vi "MoveAbsSingleAxis.vi"(6 "Wait":bool=TRUE, 8 "error in (no error)":errorcluster caption="entrée d'erreur (pas d'erreur)", 9 "Value":dbl format="%.2f", 10 "Axis":i32=1, 11 "DelayLineLS4 en entrée":refnum<class "DLLS4.lvclass">) -> (0 "error out":errorcluster caption="sortie d'erreur", 3 "DelayLineLS4 en sortie":refnum<class "DLLS4.lvclass">)   [LabVIEW 2015, in "DLLS4.lvclass"]
uses:
  DLLS4.lvclass
  DelayLine.lvclass/DelayLine.ctl
  <vilib>/Utility/error.llb/DialogType.ctl
  DelayLine.lvclass
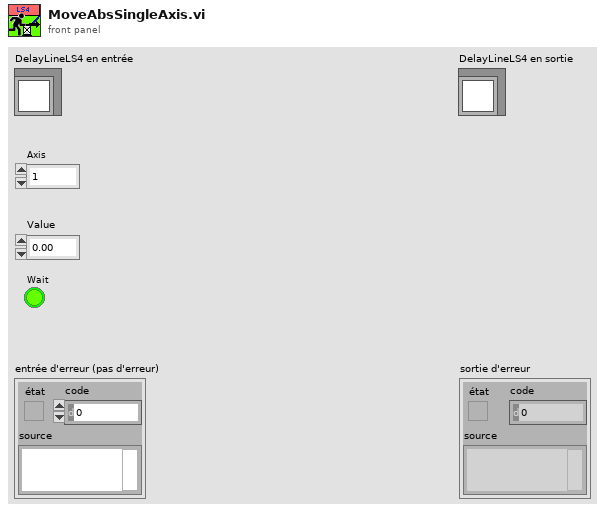
[diagram p1: front panel]
types:
  T1 = typedef "DialogType.ctl" = u16
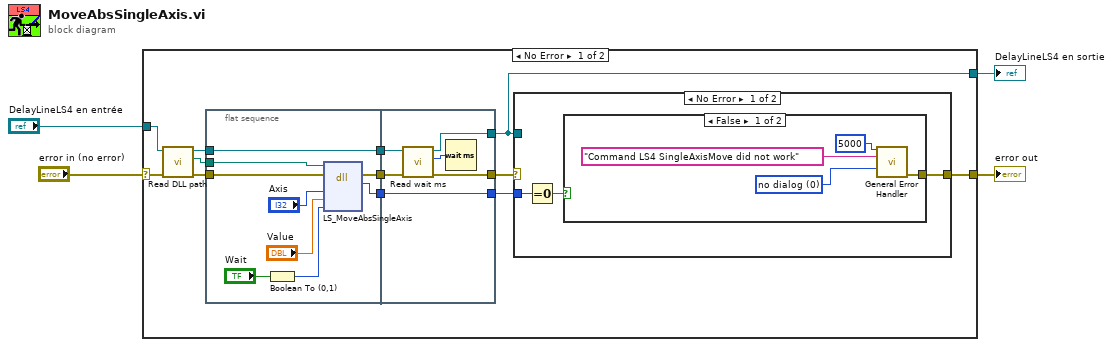
[diagram p0: block diagram]
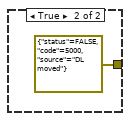
[diagram p2: hidden frame]
diagram:
  n1 = case shown="No Error" "error in (no error)" {
    selector: "error in (no error)" -> [w15 w42]
    tunnel: [w16 w42] -> w2
    tunnel: [w9 w41] -> w1
    tunnel: "DelayLineLS4 en entrée" -> [w12 w41]
    frame No Error {
      n2 = call "Read DLL path.vi"("error in (no error)"=w15, "DelayLine in"=w12) -> ("error out"=w14:errorcluster, "DLL path"=w13:path, "DelayLine out"=w11:refnum<class "DLLS4.lvclass">)  [unwired: 7 in]
      n3 = flat-sequence {
        tunnel: w14 -> [w26]
        tunnel: w13 -> [w30]
        tunnel: w11 -> [w29]
        tunnel: [w29] -> w10
        tunnel: [w28] -> w8
        tunnel: [w27] -> w6
        tunnel: [w37] -> w9
        tunnel: w10 -> [w38]
        tunnel: [w35] -> w7
        tunnel: w8 -> [w39]
        tunnel: [w40] -> w5
        tunnel: w6 -> [w40]
        frame #0 {
          n4 = Boolean To (0,1)(Boolean="Wait") -> (0, 1=w32:i16)
          n5 = dll-call lib="S:/TRANCON/DLL/LStep4.dll" fn="LS_MoveAbsSingleAxis"(path in=w30, error in=w26, "Axis"="Axis", "Value"="Value", "Wait"=w32) -> (error out=w28:errorcluster, "type de retour"=w27:i32)  [unwired: 4 in, 1 out]
        }
        frame #1 {
          n6 = call "Read wait ms.vi"("error in (no error)"=w39, "DelayLine in"=w38) -> ("error out"=w35:errorcluster, "wait ms"=w36:i32, "DelayLine out"=w37:refnum<class "DLLS4.lvclass">)  [unwired: 7 in]
          n7 = Wait (ms)(milliseconds to wait=w36) -> ()  [unwired: 1 out]
        }
      }
      n8 = case shown="No Error" w7 {
        selector: w7 -> [_ w25]
        tunnel: w5 -> [w19 _]
        tunnel: [w17 w25] -> w16
        tunnel: w9 -> [_ _]
        frame No Error {
          n9 = Equal To 0?(x=w19) -> (x = 0?=w18:bool)
          n10 = case shown="False" w18 {
            tunnel: [w20 errorcluster {"status"=FALSE, "code"=5000, "source"="DL moved"} ("error constant")] -> w17
            frame False {
              w21 = T1 0 items=["no dialog", "OK message", "continue or stop message", "OK message + warnings", "continue/stop + warnings"] ("type of dialog (OK msg:1)")
              n11 = call <vilib>:"General Error Handler.vi"("[error code] (0)"=5000 ("code"), "[error source] (\" \")"="Command LS4 SingleAxisMove did not work" ("String to Prepend to source (\"\")"), "type of dialog (OK msg:1)"=w21) -> ("error out"=w20:errorcluster)  [unwired: 8 in, 4 out]
            }
            frame True {
            }
          }
        }
        frame Error {
        }
      }
    }
    frame Error {
    }
  }
  "error out" <- w2
  "DelayLineLS4 en sortie" <- w1
